vi "armctrl-select-setpoint.vi"(6 "Set 180":bool, 8 "Set 135":bool, 9 "Set 90":bool, 10 "Set 45":bool, 11 "Set 0":bool) -> (1 "Degrees":dbl, 3 "Radians":dbl, 5 "Radian SP":T1)   [LabVIEW 2019]
uses:
  <vilib>/Analysis/Matrix/Datatypes/RealMatrix.ctl
  <vilib>/Rock Robotics/WPI/ThirdParty/JAS_Junk/TrajLib/MatBuilder_Create.vi
  <vilib>/Rock Robotics/WPI/ThirdParty/JAS_Junk/TrajLib/Trajectory_Library.lvlib
  <vilib>/Analysis/Matrix/NI_Matrix.lvlib
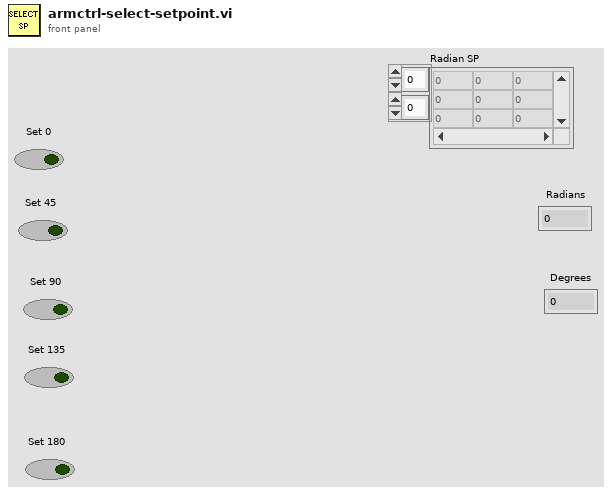
[diagram p1: front panel]
types:
  T1 = typedef "NI_Matrix.lvlib/RealMatrix.ctl" = dbl[][]
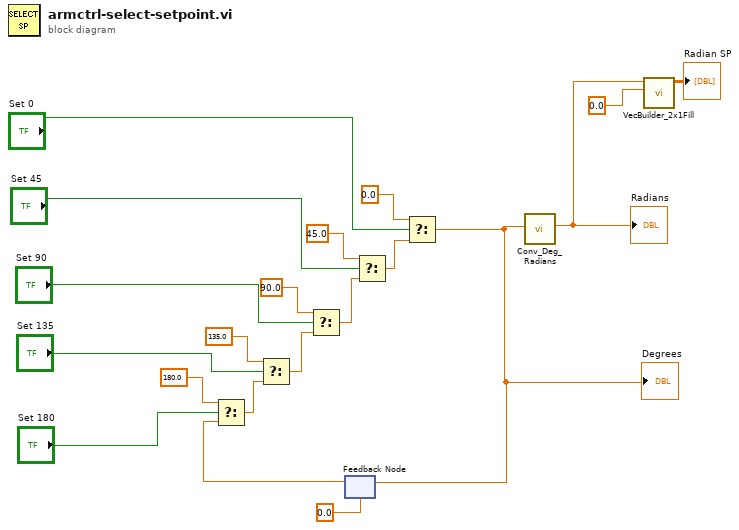
[diagram p0: block diagram]
diagram:
  n1 = feedback #1(0.0 ("t")) -> (w10:dbl)
  n2 = Select(t=180.0, s="Set 180", f=w10) -> (s? t:f=w12:dbl)
  n3 = Select(t=135.0, s="Set 135", f=w12) -> (s? t:f=w13:dbl)
  n4 = Select(t=90.0, s="Set 90", f=w13) -> (s? t:f=w14:dbl)
  n5 = Select(t=45.0, s="Set 45", f=w14) -> (s? t:f=w15:dbl)
  n6 = Select(t=0.0, s="Set 0", f=w15) -> (s? t:f=w4:dbl)
  "Degrees" <- w4
  n7 = feedback-in #1(w4) -> ()
  n8 = call <vilib>:"Conv_Deg_Radians.vi"("Degress"=w4) -> ("Radians"=w2:dbl)  [unwired: 10 in]
  "Radians" <- w2
  n9 = call <vilib>:"VecBuilder_2x1Fill.vi"("R1"=0.0, "R0"=w2) -> ("output matrix"=→"Radian SP":T1)  [unwired: 9 in]
